vi "LuaVIEW Register Public Function Directory.vi"(7 "base path":path, 11 "error in (no error)":errorcluster) -> (15 "error out":errorcluster)   [LabVIEW 2012]
doc: "Tries to register all VIs ending in \"_lua.vi\" in a directory or llb and, recursively, in any subdirectories or llbs, or, alternatively, inside a built executable as public LuaVIEW functions."
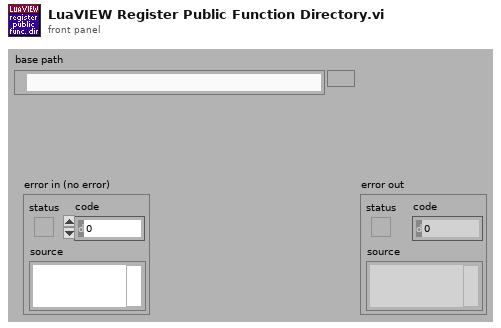
[diagram p1: front panel]
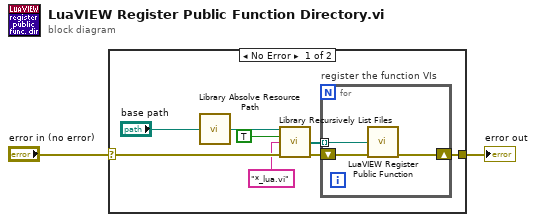
[diagram p0: block diagram]
diagram:
  n1 = case shown="No Error" "error in (no error)" {
    selector: "error in (no error)" -> [w8 w14]
    tunnel: [w7 w14] -> w2
    frame No Error {
      n2 = call "Library Absolve Resource Path.vi"("path in"="base path") -> ("absolved path"=w5:path)  [unwired: 14 in]
      n3 = call "Library Recursively List Files.vi"("root directory"=w5, "enter llbs? (no)"=TRUE, "pattern (none)"="*_lua.vi" ("pattern"), "error in (no error)"=w8) -> ("file list"=w10:path[], "error out"=w9:errorcluster)  [unwired: 9 in, 1 out]
      n4 = for "register the function VIs" {
        shift-right: [w12] -> w7
        shift-left: w9 -> [w13]
        tunnel: w10 -> [w11] mode=indexing
        n5 = call "LuaVIEW Register Public Function.vi"("function VI path"=w11, "error in (no error)"=w13) -> ("error out"=w12:errorcluster)  [unwired: 13 in]
      }
    }
    frame Error {
    }
  }
  "error out" <- w2
